vi "getInputParameter.vi"(8 "error in (no error)":errorcluster, 11 "HGF_Visitable.lvclass in":refnum<class "HGF_Visitable.lvclass">) -> (0 "error out":errorcluster, 2 "input":variant, 3 "HGF_Visitable.lvclass out":refnum<class "HGF_Visitable.lvclass">)   [LabVIEW 2014, in "HGF_BaseClasses.lvlib" / "HGF_Visitable.lvclass"]
doc: "get input parameter attribute."
uses:
  HGF_Visitable.lvclass
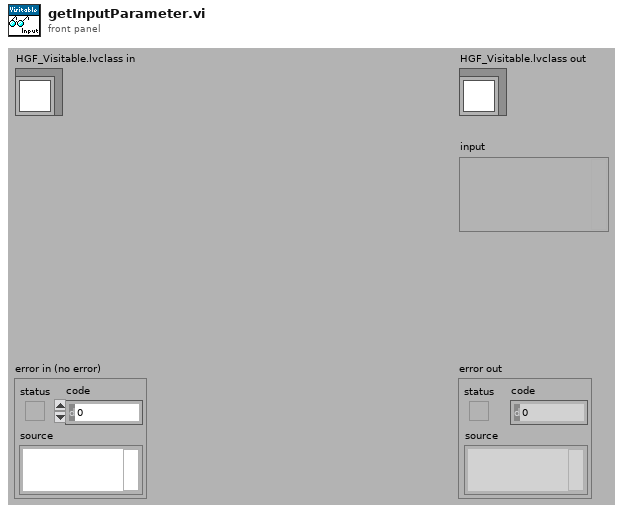
[diagram p1: front panel]
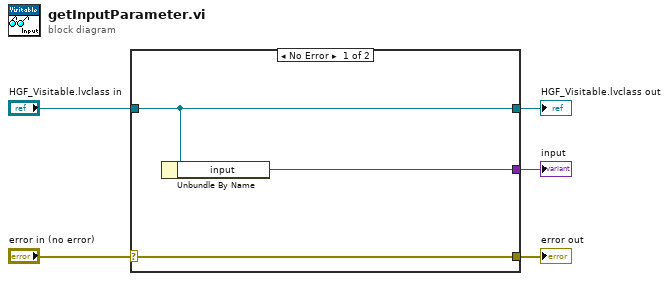
[diagram p0: block diagram]
diagram:
  n1 = case shown="No Error" "error in (no error)" {
    selector: "error in (no error)" -> [w8 w9]
    tunnel: [w8 w9] -> w4
    tunnel: [w7 w10] -> w2
    tunnel: "HGF_Visitable.lvclass in" -> [w7 w10]
    tunnel: [w6 _] -> w1
    frame No Error {
      n2 = Unbundle By Name(w7) -> ("input"=w6:variant)
    }
    frame Error {
    }
  }
  "error out" <- w4
  "HGF_Visitable.lvclass out" <- w2
  "input" <- w1
